vi "SIMPLE_Read_Config.vi"() -> ()   [LabVIEW 2016]
uses:
  <vilib>/Instr/_visa.llb/VISA Set IO Buffer Mask.ctl
  <vilib>/Utility/miscctls.llb/LVPointTypeDef.ctl
  <vilib>/Instr/_visa.llb/VISA Configure Serial Port (Instr).vi
  REV_2.lvlib
  REV2_Config_Addr.ctl
panel:
  out "Error count":u64
  in  "Address":T1[](array[typedef])=[2, 1, 27, 28] items=["ID", "Mode", "Baudrate", "Homing Offset", "Id P gain", "Id I gain", "Id D gain", "Iq P gain", "Iq I gain", "Iq D gain", "Velo P gain", "Velo I gain", "Velo D gain", "Posi P gain", "Posi I gain", "Posi D gain", "DirectForce P", "DirectForce I", "DirectForce D", "Limit Id Max", "Limit Iq Max", "Limit Velo Max", "Limit Posi Min", "Limit Posi Max", "Voltage Min", "Voltage Max", "Watchdog", "Temperature Low", "Temperature High"]
  out "ERROR":u8
  out "value":dbl[](array[numeric])=[8000000.0, 3.0, 80.0, 100.0]
  in  "ID":u8=1 format="%x"
  in  "Read":bool
  in  "Baud rate":u32=8000000
  in  "Com port":refnum<visa-resource-name>="COM15"
  in  "stop":bool
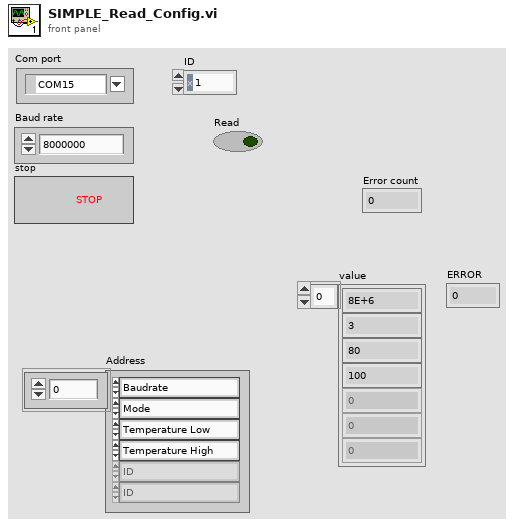
[diagram p1: front panel]
types:
  T1 = typedef "REV_2.lvlib/REV2_Config_Addr.ctl" = u8
  T2 = typedef "LVPointTypeDef.ctl" = cluster{"Horizontal":i16, "Vertical":i16}
  T3 = typedef "VISA Set IO Buffer Mask.ctl" = u16
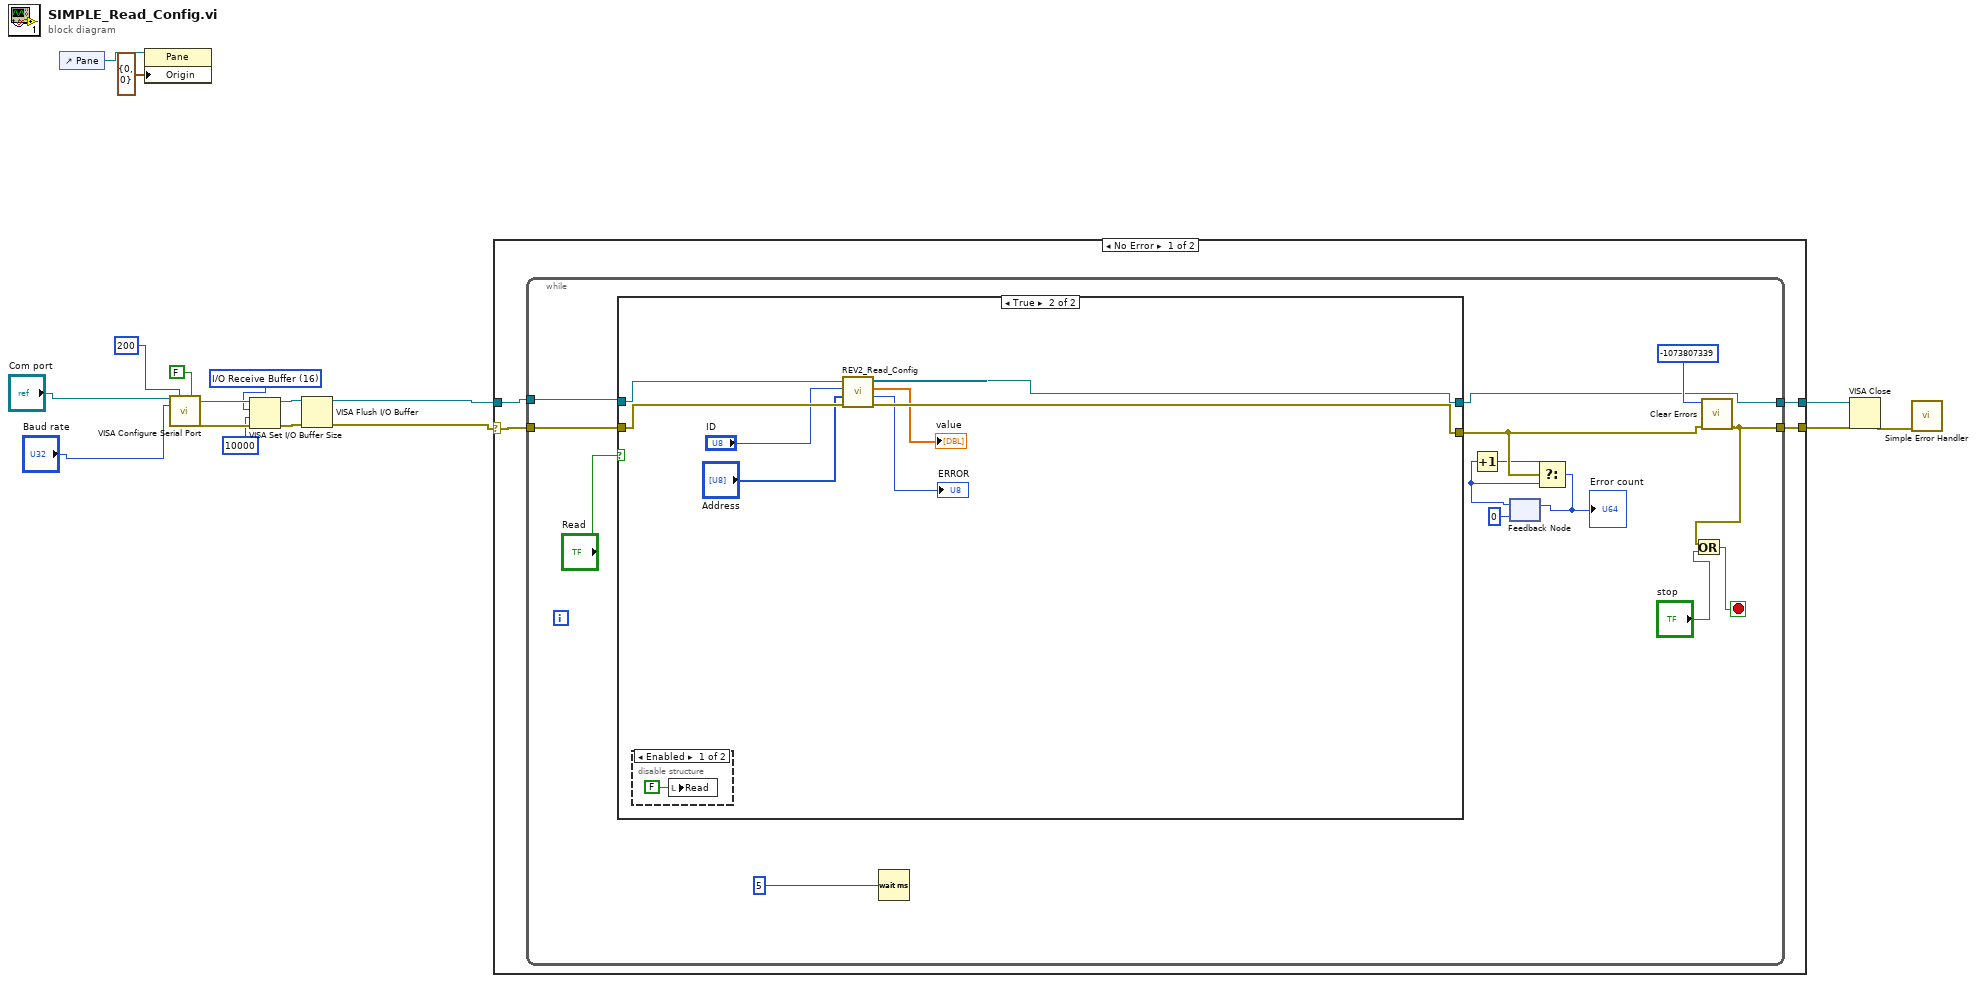
[diagram p0: block diagram]
diagram:
  w9 = T3 16 items=["I/O Receive Buffer"=16, "I/O Transmit Buffer"=32, "I/O Receive and Transmit Buffer"=48] ("Mask")
  n1 = control-ref of="Pane"() -> (w4:refnum<vi>)
  n2 = property class="Pane"(reference=w4, "Origin"=T2 {"Horizontal"=0, "Vertical"=0}) -> ()  [unwired: 1 in, 2 out]
  n3 = call-poly "VISA Configure Serial Port"("VISA resource name"="Com port", "timeout (10sec)"=u32 200, "Enable Termination\nChar (T)"=FALSE ("Enable Termination\nChar (T)"), "baud rate (9600)"="Baud rate") -> ("VISA resource name out"=w10:refnum<visa-resource-name>, "error out"=w13:errorcluster)  [unwired: 10 in]
  n4 = VISA Set I/O Buffer Size(VISA resource name=w10, mask (16)=w9, size (4096)=u32 10000, error in (no error)=w13) -> (VISA resource name out=w11:refnum<visa-resource-name>, error out=w12:errorcluster)
  n5 = VISA Flush I/O Buffer(VISA resource name=w11, error in (no error)=w12) -> (VISA resource name out=w1:refnum<visa-resource-name>, error out=w2:errorcluster)  [unwired: 1 in]
  n6 = case shown="No Error" w2 {
    selector: w2 -> [w18 w47]
    tunnel: [w21 w47] -> w17
    tunnel: w1 -> [w20 w48]
    tunnel: [w19 w48] -> w15
    frame No Error {
      n7 = while {
        tunnel: w20 -> [w31]
        tunnel: w18 -> [w30]
        tunnel: [w28] -> w19
        tunnel: [w29] -> w21
        stop <- w34 stop-if-true
        n8 = case shown="True" "Read" {
          tunnel: w30 -> [w37 w45]
          tunnel: w31 -> [w36 w44]
          tunnel: [w36 w41] -> w28
          tunnel: [w37 w42] -> w25
          frame False {
          }
          frame True {
            n9 = disable-structure shown="Enabled" {
              frame Enabled {
                n10 = local write "Read"(FALSE ("write")) -> ()
              }
              frame Disabled {
              }
            }
            n11 = call "REV2_Read_Config.vi"("error in (no error)"=w45, "Config Address"="Address", "ID"="ID", "VISA Refnum in"=w44) -> ("error out"=w42:errorcluster, "ERROR"=→"ERROR":u8, "Data"=→"value":dbl[], "VISA Refnum out"=w41:refnum<visa-resource-name>)  [unwired: 4 in]
          }
        }
        n12 = Wait (ms)(milliseconds to wait=u32 5) -> ()  [unwired: 1 out]
        n13 = feedback #1(u64 0) -> (w23:u64)
        n14 = Increment(x=w23) -> (x+1=w24:u64)
        n15 = Select(t=w24, s=w25, f=w23) -> (s? t:f=w22:u64)
        "Error count" <- w22
        n16 = feedback-in #1(w22) -> ()
        n17 = call <vilib>:"Clear Errors.vi"("error in (no error)"=w25, "specific error code to clear (0: all)"=-1073807339) -> ("error out"=w29:errorcluster)  [unwired: 4 in, 1 out]
        n18 = Or(x=w29, y="stop") -> (x .or. y?=w34:bool)
      }
    }
    frame Error {
    }
  }
  n19 = VISA Close(VISA resource name=w15, error in (no error)=w17) -> (error out=w7:errorcluster)
  n20 = call <vilib>:"Simple Error Handler.vi"("error in (no error)"=w7) -> ()  [unwired: 4 in, 5 out]
